vi "mod0.vi"() -> (0 "new picture":picture)   [LabVIEW 2010]
panel:
  in  "Stopp":bool
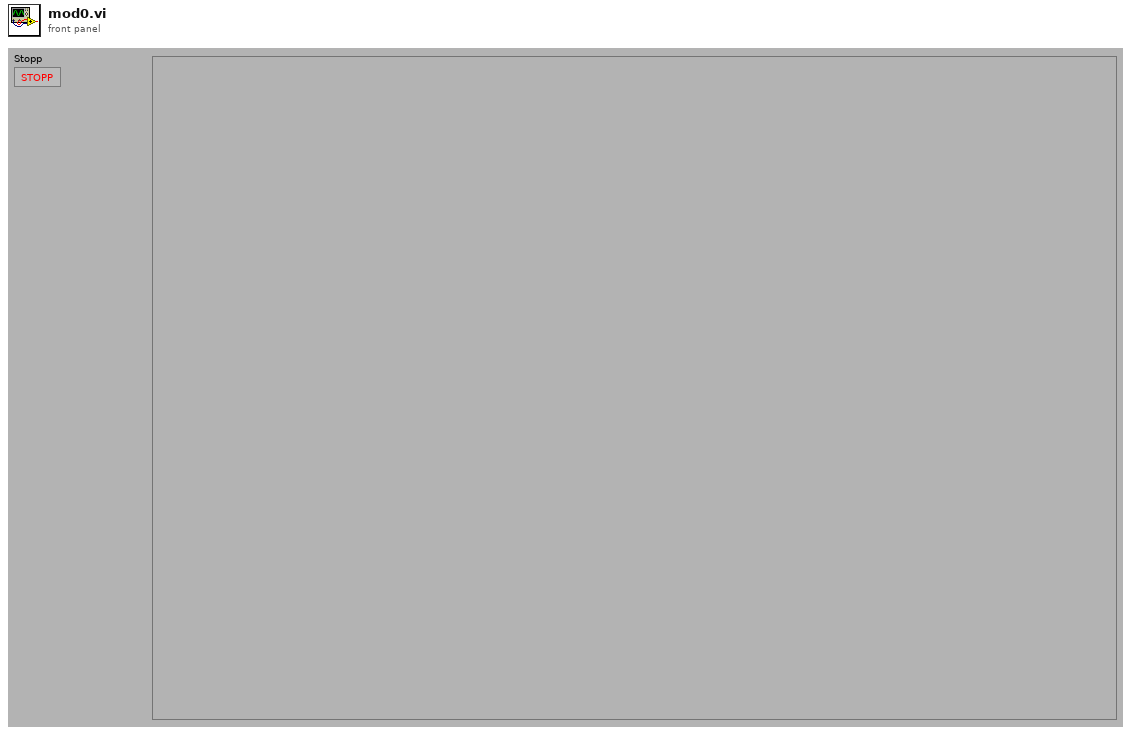
[diagram p1: front panel]
types:
  T1 = typedef "imagedata.ctl" = cluster{"image type":i32, "image depth":i32, "image":u8[], "mask":u8[], "colors":u32[], "Rectangle":cluster{"left":i16, "top":i16, "right":i16, "bottom":i16}}
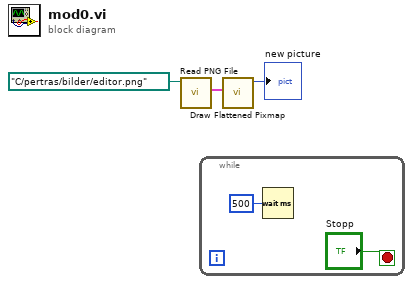
[diagram p0: block diagram]
diagram:
  n1 = call <vilib>:"Read PNG File.vi"("path to PNG file"=path "C:/pertras/bilder/editor.png") -> ("image data"=w3:T1)  [unwired: 8 in, 2 out]
  n2 = while {
    stop <- "Stopp" stop-if-true
    n3 = Wait (ms)(milliseconds to wait=u32 500 ("Zu wartende ms")) -> ()  [unwired: 1 out]
  }
  n4 = call <vilib>:"Draw Flattened Pixmap.vi"("image data"=w3) -> ("new picture"=→"new picture":picture)  [unwired: 8 in]
